vi "ButtonDropOpen.vi"(11 "Buttons":bool[](array[boolean])) -> (3 "Boolean":bool)   [LabVIEW 2014]
uses:
  Gantry/GantryGlobals.vi
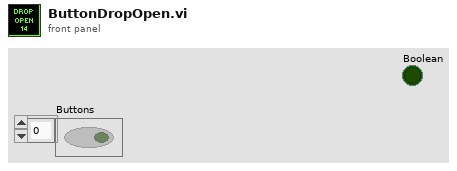
[diagram p1: front panel]
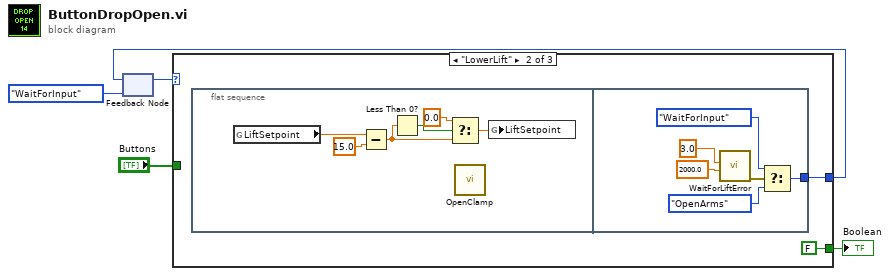
[diagram p0: block diagram]
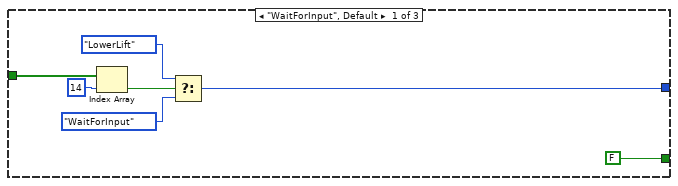
[diagram p2: hidden frame]
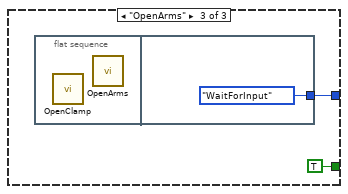
[diagram p3: hidden frame]
diagram:
  n1 = feedback #1(enum16{"WaitForInput", "LowerLift", "OpenArms"}."WaitForInput" ("Enum")) -> (w4:enum16{"WaitForInput", "LowerLift", "OpenArms"})
  n2 = case shown="\"LowerLift\"" w4 {
    tunnel: [w11 w14 w28] -> w3
    tunnel: "Buttons" -> [w10 _ _]
    tunnel: [FALSE FALSE TRUE] -> w1
    frame "WaitForInput", Default {
      n3 = Index Array(array=w10, index=14) -> (element=w7:bool)
      n4 = Select(t=enum16{"WaitForInput", "LowerLift", "OpenArms"}."LowerLift" ("Enum"), s=w7, f=enum16{"WaitForInput", "LowerLift", "OpenArms"}."WaitForInput" ("Enum")) -> (s? t:f=w11:enum16{"WaitForInput", "LowerLift", "OpenArms"})
    }
    frame "LowerLift" {
      n5 = flat-sequence {
        tunnel: [w23] -> w14
        frame #0 {
          n6 = global read "GantryGlobals.vi" "LiftSetpoint"() -> (w20:dbl)
          n7 = Subtract(x=w20, y=15.0) -> (x-y=w16:dbl)
          n8 = Less Than 0?(x=w16) -> (x < 0?=w18:bool)
          n9 = Select(t=0.0, s=w18, f=w16) -> (s? t:f=w15:dbl)
          n10 = call "OpenClamp.vi"() -> ()  [unwired: 12 in]
          n11 = global write "GantryGlobals.vi" "LiftSetpoint"(w15) -> ()
        }
        frame #1 {
          n12 = call "WaitForLiftError.vi"("Timeout (ms)"=2000.0, "AllowedError"=3.0) -> ("error out"=w26:errorcluster)  [unwired: 9 in]
          n13 = Select(t=enum16{"WaitForInput", "LowerLift", "OpenArms"}."WaitForInput" ("Enum"), s=w26, f=enum16{"WaitForInput", "LowerLift", "OpenArms"}."OpenArms" ("Enum")) -> (s? t:f=w23:enum16{"WaitForInput", "LowerLift", "OpenArms"})
        }
      }
    }
    frame "OpenArms" {
      n14 = flat-sequence {
        tunnel: [enum16{"WaitForInput", "LowerLift", "OpenArms"}."WaitForInput" ("Enum")] -> w28
        frame #0 {
          n15 = call "OpenClamp.vi"() -> ()  [unwired: 12 in]
          n16 = call "OpenArms.vi"() -> ()  [unwired: 12 in]
        }
        frame #1 {
        }
      }
    }
  }
  "Boolean" <- w1
  n17 = feedback-in #1(w3) -> ()
